vi "Analog Output Scan.vi"(8 "error in (no error)":errorcluster, 10 "Analog Output.lvclass":refnum<class "Analog Output.lvclass">, 11 "Analog Out Scan in":refnum<class "Analog Output Scan.lvclass">) -> (0 "error out":errorcluster, 3 "Analog Out Scan out":refnum<class "Analog Output Scan.lvclass">)   [LabVIEW 2017, in "Analog Output Scan.lvclass"]
uses:
  Analog Output Scan.lvclass
  C:/LabVIEW-programs/Scanners/Scanner/Scanner.lvclass
  Instruments/Analog Output/Analog Output.lvclass
  C:/LabVIEW-programs/Instruments/Utility Classes/Scannable/Scannable.lvclass
  Scanner/Scanner.lvclass
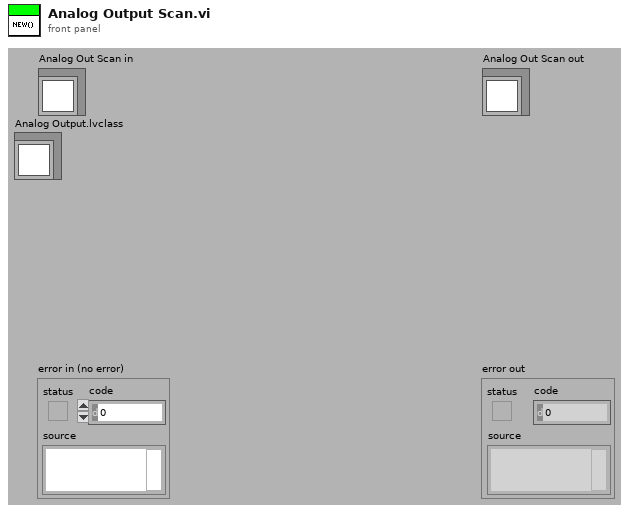
[diagram p1: front panel]
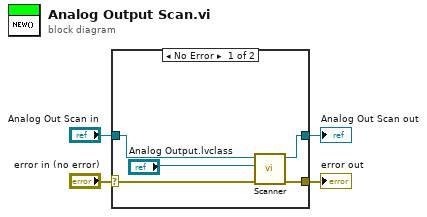
[diagram p0: block diagram]
diagram:
  n1 = case shown="No Error" "error in (no error)" {
    selector: "error in (no error)" -> [w7 w11]
    tunnel: [w6 w11] -> w3
    tunnel: [w8 w10] -> w1
    tunnel: "Analog Out Scan in" -> [w9 w10]
    frame No Error {
      n2 = call "Scanner.vi"("error in (no error)"=w7, "Scannable"="Analog Output.lvclass", "Scanner.lvclass in"=w9) -> ("error out"=w6:errorcluster, "Scanner.lvclass out"=w8:refnum<class "Analog Output Scan.lvclass">)  [unwired: 1 in, 6 out]
    }
    frame Error {
    }
  }
  "error out" <- w3
  "Analog Out Scan out" <- w1
